vi "Transport.vi"(4 "Queue of Error":refnum<queue>, 6 "Queue of Self Attributes":refnum<queue>, 7 "Actor in":refnum<class "Actor.lvclass">, 10 "Attributes":refnum<class "Attributes.lvclass">) -> (0 "Error out":errorcluster, 5 "Actor out":refnum<class "Actor.lvclass">)   [LabVIEW 2025, in "jettl.lvlib" / "Transport.lvlib" / "Queue.lvlib"]
uses:
  Queue.lvlib
  Actor/Actor.lvclass
  Attributes/Attributes/Attributes.lvclass
  Msg Output/Msg Output.lvclass
  jettl.lvlib
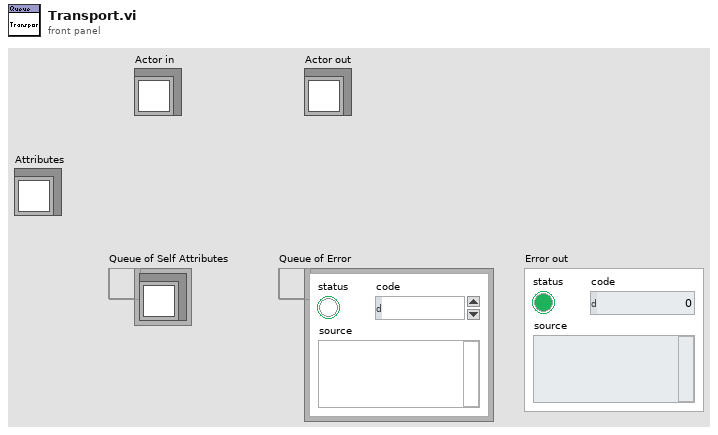
[diagram p1: front panel]
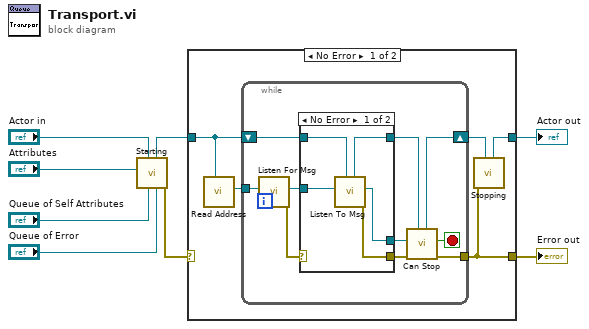
[diagram p0: block diagram]
diagram:
  n1 = call "Starting.vi"("Queue of Error"="Queue of Error", "Queue of Self Attributes"="Queue of Self Attributes", "Actor in"="Actor in", "Attributes"="Attributes") -> ("Error out"=w1:errorcluster, "Actor out"=w6:refnum<class "Actor.lvclass">)  [unwired: 6 in]
  n2 = case shown="No Error" w1 {
    selector: w1 -> [_ w32]
    tunnel: [w11 w31] -> w7
    tunnel: [w13 w32] -> w8
    tunnel: w6 -> [w9 w31]
    frame No Error {
      n3 = call "Read Address.vi"("Actor"=w9) -> ("Address"=w10:refnum<data-value>)  [unwired: 10 in]
      n4 = while {
        shift-right: [w21] -> w12
        shift-left: w9 -> [w19]
        tunnel: [w22] -> w13
        tunnel: w10 -> [w17]
        stop <- w20 stop-if-true
        n5 = call "Listen For Msg.vi"("Address"=w17) -> ("Error out"=w15:errorcluster, "Msg"=w16:refnum<class "Msg.lvclass">)  [unwired: 9 in]
        n6 = case shown="No Error" w15 {
          selector: w15 -> [_ w29]
          tunnel: [w25 w29] -> w23
          tunnel: w19 -> [w28 w30]
          tunnel: [w26 w30] -> w18
          tunnel: w16 -> [w27 _]
          tunnel: [w24 _] -> w14
          frame No Error {
            n7 = call "Listen To Msg.vi"("Actor in"=w28, "Msg"=w27) -> ("Error out"=w25:errorcluster, "Msg Output"=w24:refnum<class "Msg Output.lvclass">, "Actor out"=w26:refnum<class "Actor.lvclass">)  [unwired: 7 in]
          }
          frame Error {
          }
        }
        n8 = call "Can Stop.vi"("Actor in"=w18, "Error in"=w23, "Msg Output"=w14) -> ("Error out"=w22:errorcluster, "Stop"=w20:bool, "Actor out"=w21:refnum<class "Actor.lvclass">)  [unwired: 6 in]
      }
      n9 = call "Stopping.vi"("Actor in"=w12, "Error in"=w13) -> ("Actor out"=w11:refnum<class "Actor.lvclass">)  [unwired: 9 in]
    }
    frame Error {
    }
  }
  "Error out" <- w8
  "Actor out" <- w7
